vi "Reset.vi"(8 "error in (no error)":errorcluster, 11 "VISA resource name":refnum<visa-resource-name>) -> (0 "error out":errorcluster, 3 "VISA resource name out":refnum<visa-resource-name>)   [LabVIEW 2024, in "U1250 Series Digital Multimeter.lvlib"]
doc: "Resets the instrument and then sends a set of default setup commands to the instrument."
uses:
  U1250 Series Digital Multimeter.lvlib
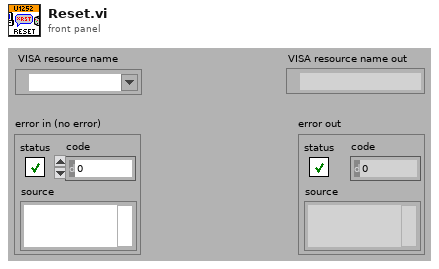
[diagram p1: front panel]
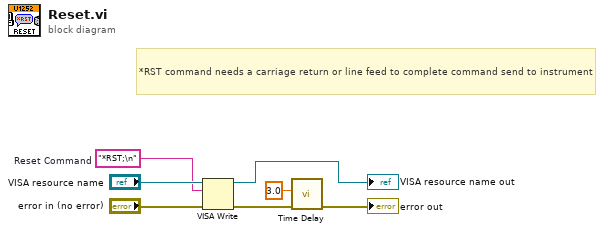
[diagram p0: block diagram]
diagram:
  w5 = "*RST;\n"  # Reset Command
  # "*RST command needs a carriage return or line feed to complete command send to instrument"
  n1 = VISA Write(VISA resource name="VISA resource name", write buffer=w5, error in (no error)="error in (no error)") -> (VISA resource name out=→"VISA resource name out":refnum<visa-resource-name>, error out=w4:errorcluster)  [unwired: 1 out]
  n2 = call "Time Delay"("error in (no error)"=w4, "Delay Time (s)"=3.0) -> ("error out"=→"error out":errorcluster)  [unwired: 9 in]
